vi "integrated_draft_1.vi"() -> ()   [LabVIEW 2014]
doc: "This VI demonstrates the individual configuration of settings in I/W, W/I, and continuous operation modes.\n\nThis VI is not meant to be used with infusion-only models. \n\nNotes:\n(1) If continuous mode is selected, infuse volumes/rates will be used."
uses:
  <vilib>/Motion/FlexMotion/CustomControls/CustomControls.llb/AxisOrVectorSpace To Configure.flx
  <vilib>/Motion/FlexMotion/FunctionsVIs/StartStopMotion.llb/Start Motion (8 axes).flx
  <vilib>/Motion/FlexMotion/FunctionsVIs/Trajectory.llb/Check Move Complete Status (8 axes).flx
  <vilib>/Motion/FlexMotion/FunctionsVIs/StartStopMotion.llb/Stop Motion (8 axes).flx
  <instrlib>/KD Scientific 2XX Series/KD Scientific 2XX Series.lvlib
  <vilib>/vision/NI_Vision_Development_Module.lvlib
panel:
  in  "stop 2":bool
  out "Voltage (V)":dbl=0.3869919147841388
  out "Force (grams)":dbl=0.3869919147841388
  out "Force Graph (g)":dynamicdata(graph)
  in  "Zero":dbl=-99.6 format="%#_13g"
  out "Load Cell Output (mV)":dynamicdata(graph)
  in  "stop (F)":bool
  out "Darta from Pressure Transducer":dynamicdata(graph) caption="data"
  out "Pressure Transducer Array":dbl[](array[numeric])
  in  "Displacement in mm":dbl
  in  "Velocity in mm/s":dbl
  out "Image":T1(plugin-control)
  out "Particle Measurements (Pixels) (Particle Analysis 1)":dbl[][](array[numeric]) format="%.2f"
  out "subarray":dbl[](array[numeric])
  out "The diameter":dbl[](array[numeric])
  out "Image from  Vision Acquisition 1":T1(plugin-control)
  out "Units":string
  out "Delivered Volume":dbl
  in  "stop":bool
  out "Status":T2
  in  "Baud Rate (9600)":u32(ring)=9600 items=["300"=300, "1200"=1200, "2400"=2400, "4800"=4800, "9600"=9600]
  in  "Withdrawal Settings":T3={"Flow Rate (5)"=5.0, "Volume (10)"=10.0, "Volume Units (ml)"=enum."milliliters (ml)", "Rate Units (ml/min.)"=enum."milliliters per minute (ml/min.)"} {"Volume (10)" format="%#.3g"}
  in  "Diameter (8.75 mm)":dbl=8.75
  in  "Infusion Settings":T3={"Flow Rate (5)"=5.0, "Volume (10)"=10.0, "Volume Units (ml)"=enum."milliliters (ml)", "Rate Units (ml/min.)"=enum."milliliters per minute (ml/min.)"}
  in  "Operation Mode (Infuse)":u16(ring) items=["Infuse", "Withdraw", "Infuse-Withdraw", "Withdraw-Infuse", "Continuous"]
  in  "Address (0)":i32 format="%0.0f"
  in  "error in (no error)":errorcluster
  in  "VISA resource name":refnum<visa-resource-name>="COM1"
  # "CCD Camera Input"
  # "Load Cell Input"
  # "Syringe Pump Control"
  # "RS-232 Settings"
  # "General Settings"
  # "Pump Status"
  # "Pressure Transducer"
  # "Displacement Motor Control"
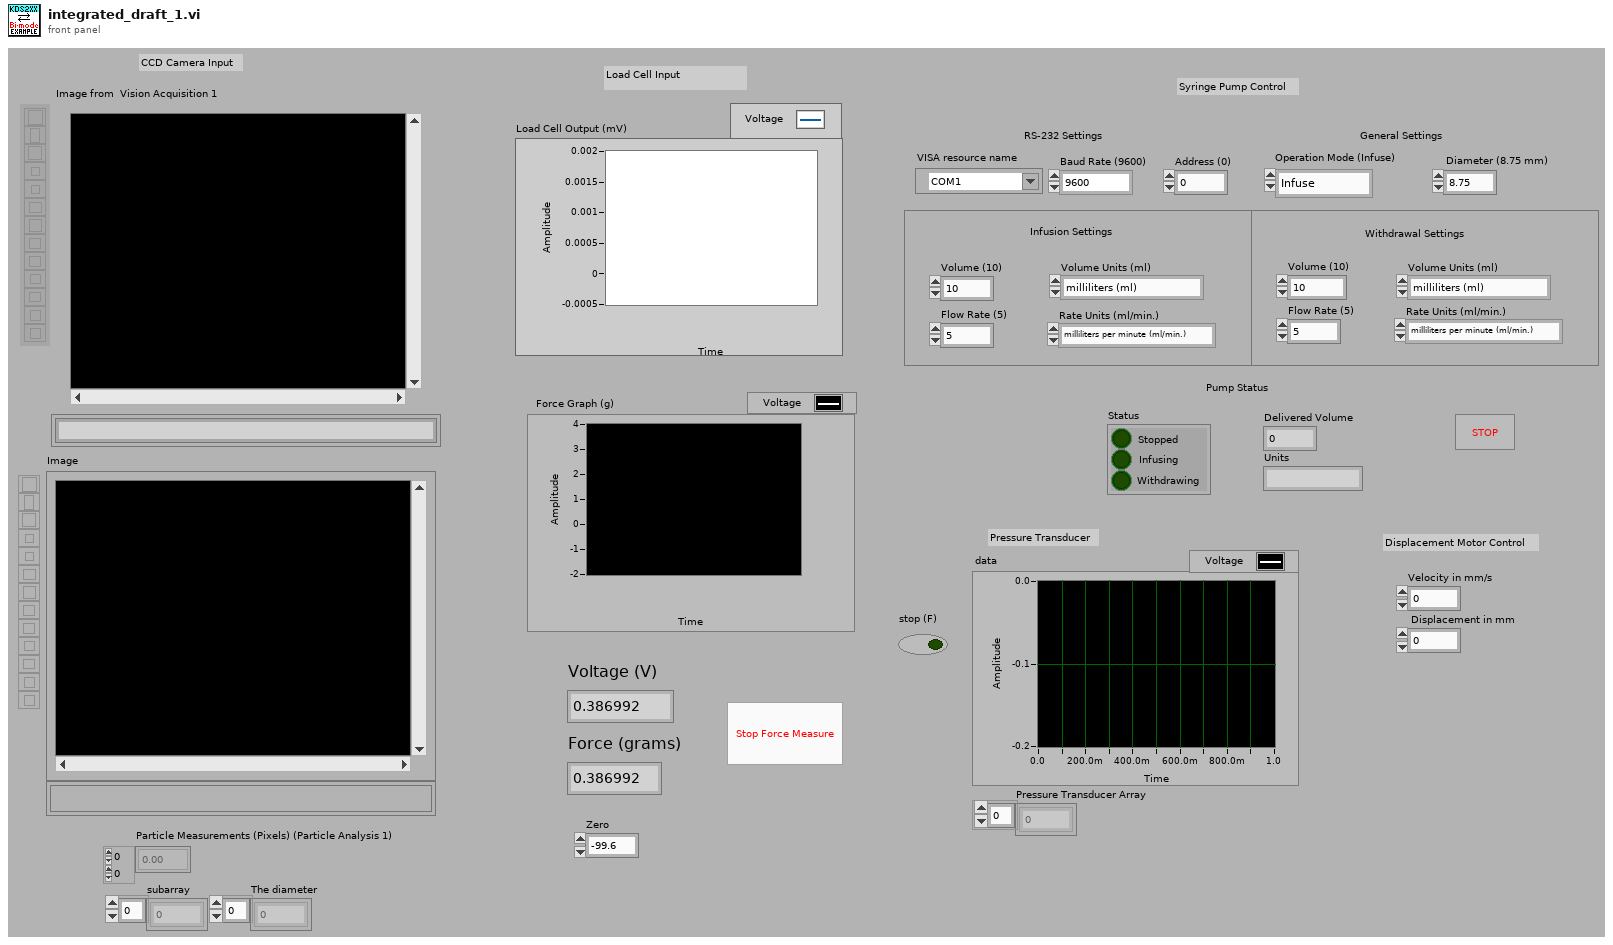
[diagram p1: front panel]
types:
  T1 = typedef "IMAQ Image.ctl" = refnum<image>
  T2 = cluster{"Stopped":bool, "Infusing":bool, "Withdrawing":bool}
  T3 = cluster{"Flow Rate (5)":dbl, "Volume (10)":dbl, "Volume Units (ml)":enum16{"milliliters (ml)", "microliters (ul)"}, "Rate Units (ml/min.)":enum16{"milliliters per minute (ml/min.)", "milliliters per hour (ml/hr.)", "microliters per minute (ul/min.)", "microliters per hour (ul/hr.)"}}
  T4 = typedef "Board Id" = u8
  T5 = enum16{"Absolute Position", "Relative Position", "Velocity", "Relative to Cap Pos", "Modulus Position", "Absolute Contouring", "Relative Contouring"}
  T6 = typedef "ROI Descriptor" = cluster{"Global Rectangle":i32[], "Contours":cluster{"ID":enum32{"External", "Internal"}, "Type":u32, "Coordinates":i32[]}[]}
  T7 = typedef "AxisOrVectorSpace To Configure.flx" = u16
  T8 = typedef "Resource Out (Enum).flx" = u16
  T9 = typedef "Bd Id Out" = u8
  T10 = enum16{"milliliters per minute (ml/min.)", "milliliters per hour (ml/hr.)", "microliters per minute (ul/min.)", "microliters per hour (ul/hr.)"}
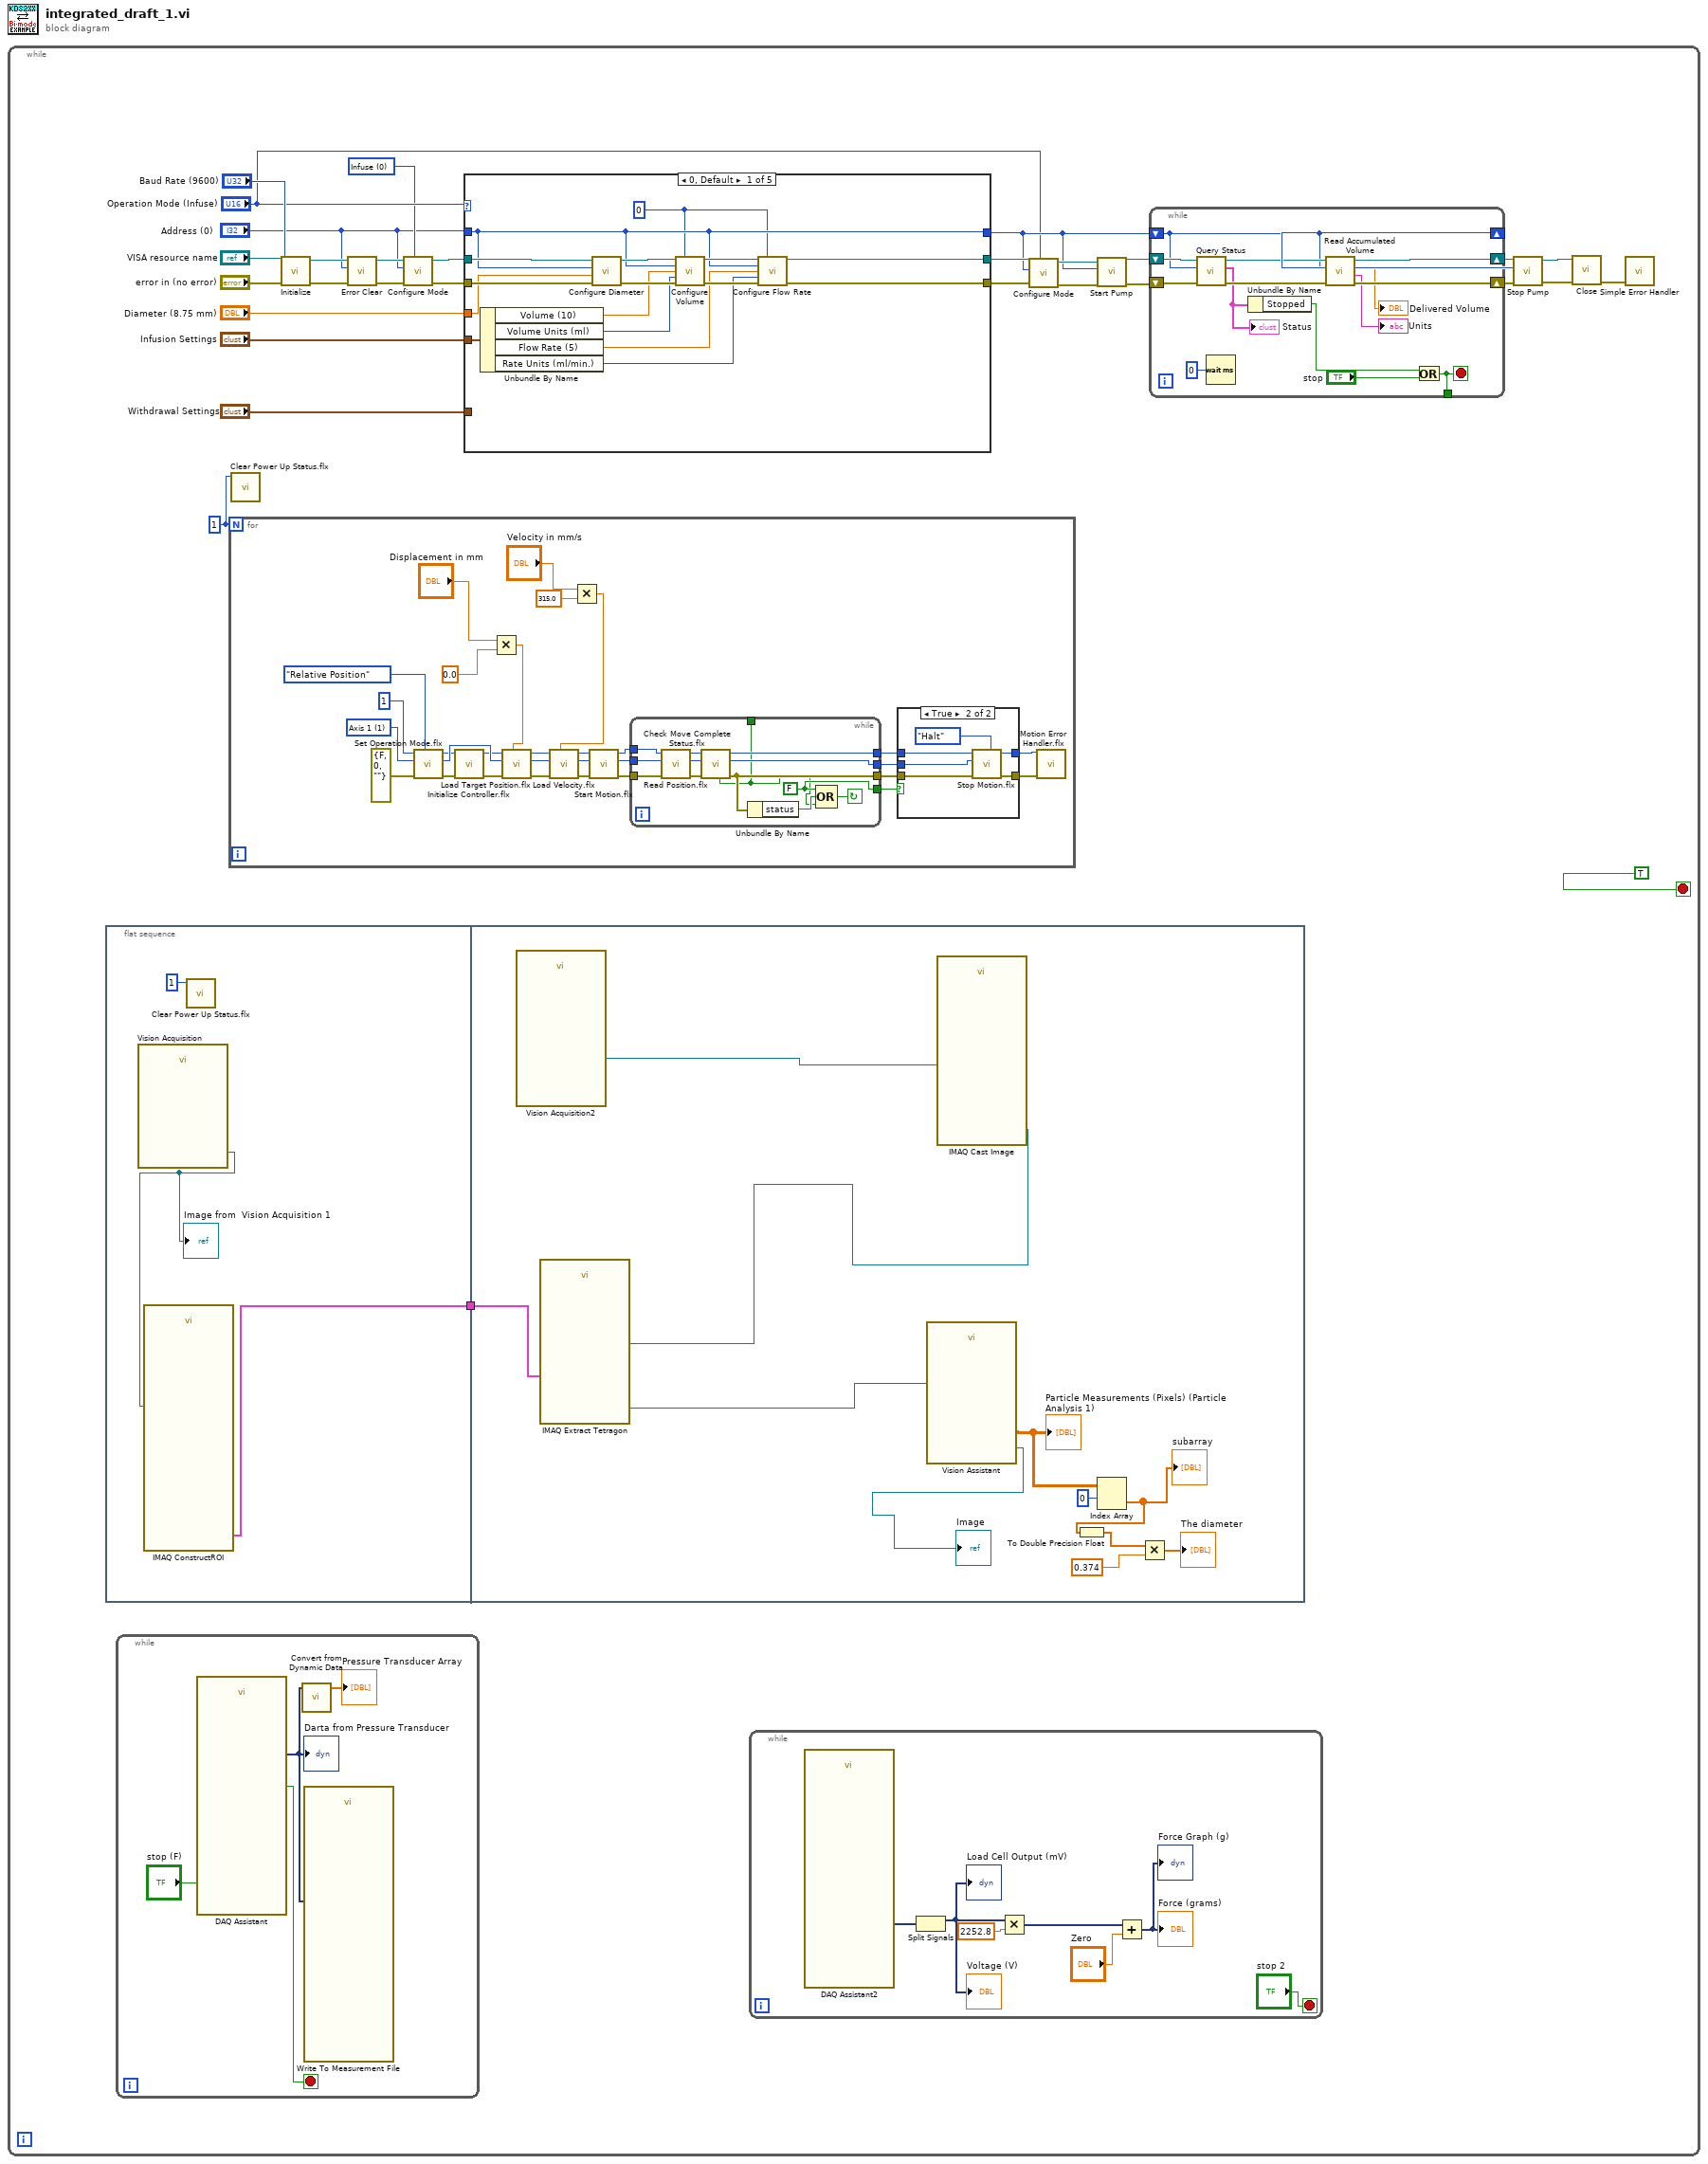
[diagram p0: block diagram]
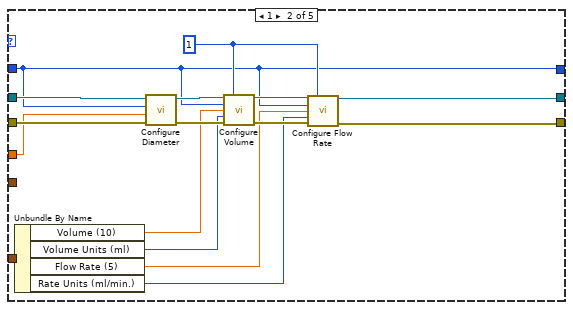
[diagram p3: hidden frame]
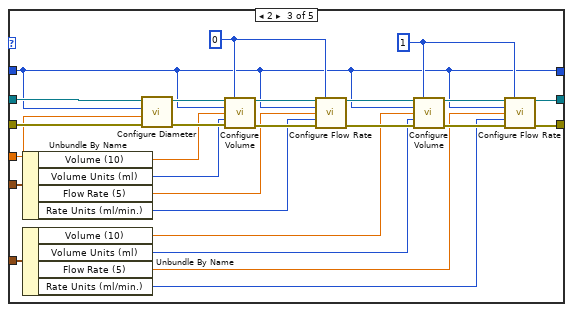
[diagram p4: hidden frame]
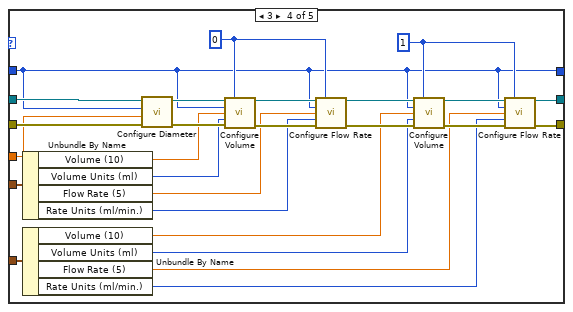
[diagram p5: hidden frame]
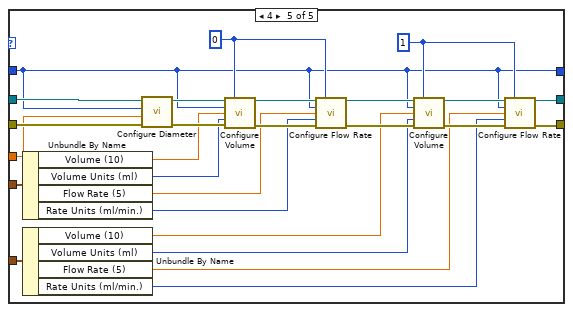
[diagram p6: hidden frame]
diagram:
  n1 = while {
    stop <- TRUE stop-if-true
    w3 = T4 1 ("Board ID")
    w9 = u16 0 items=["Infuse", "Withdraw", "Infuse-Withdraw", "Withdraw-Infuse", "Continuous"] ("Mode (infuse)")
    n2 = flat-sequence {
      tunnel: [w45] -> w1
      tunnel: w1 -> [w56]
      frame #0 {
        n3 = call "Vision Acquisition"() -> ("Image Out"=w43:T1)  [unwired: 26 in, 1 out]
        "Image from  Vision Acquisition 1" <- w43
        n4 = call "IMAQ ConstructROI"("Image"=w43) -> ("ROI Descriptor Out"=w45:T6)  [unwired: 7 in, 3 out]
        n5 = call <vilib>:"Clear Power Up Status.flx"("Board ID"=T4 1) -> ()  [unwired: 6 in, 2 out]
      }
      frame #1 {
        n6 = call "Vision Acquisition2"() -> ("Image Out"=w54:T1)  [unwired: 25 in, 2 out]
        n7 = call "IMAQ Cast Image"("Image Src"=w54) -> ("Image Dst Out"=w52:T1)  [unwired: 9 in, 1 out]
        n8 = call-poly "IMAQ Extract Tetragon"("ROI Descriptor"=w56, "Image Src"=w52) -> ("Image Dst Out"=w53:T1)  [unwired: 8 in, 1 out]
        n9 = call "Vision Assistant"("Image In"=w53) -> ("Image Out"=→"Image":T1, "Particle Measurements (Pixels) (Particle Analysis 1)"=w51:dbl[][])  [unwired: 23 in, 2 out]
        "Particle Measurements (Pixels) (Particle Analysis 1)" <- w51
        n10 = Index Array(array=w51, index (row)=0) -> (element=w49:dbl[])  [unwired: 1 in]
        "subarray" <- w49
        n11 = To Double Precision Float(number=w49) -> (double precision float=w48:dbl[])
        n12 = Multiply(x=w48, y=0.374) -> (x*y=→"The diameter":dbl[])
      }
    }
    n13 = while {
      stop <- w41 stop-if-true
      n14 = call "DAQ Assistant"("stop (F)"="stop (F)") -> ("data"=w39:dynamicdata, "stopped"=w41:bool)  [unwired: 15 in, 2 out]
      "Darta from Pressure Transducer" <- w39
      n15 = call "Convert from Dynamic Data"("Dynamic Data Type"=w39) -> ("Array"=→"Pressure Transducer Array":dbl[])  [unwired: 3 in]
      n16 = call "Write To Measurement File"("Signals"=w39) -> ()  [unwired: 16 in, 3 out]
    }
    n17 = for {
      N: w3 -> [_]
      w84 = T7 1 items=["Axis 1"=1, "Axis 2"=2, "Axis 3"=3, "Axis 4"=4, "Axis 5"=5, "Axis 6"=6, "Axis 7"=7, "Axis 8"=8, "Vector Space 1"=17, "Vector Space 2"=18, "Vector Space 3"=19, "Vector Space 4"=20] ("Axis or Vector Space")
      n18 = call <vilib>:"Set Operation Mode.flx"("Position Mode (Absolute)"=T5."Relative Position", "error in (no error)"=errorcluster {"status"=FALSE, "code"=0, "source"=""} ("error constant"), "Axis or Vector Space"=w84, "Board ID"=T4 1) -> ("error out"=w82:errorcluster, "Resource Output"=w81:T8, "Bd ID Out"=w80:T9)  [unwired: 2 in]
      n19 = call <vilib>:"Initialize Controller.flx"("error in (no error)"=w82, "Board ID"=w80) -> ("error out"=w75:errorcluster, "Bd ID Out"=w79:T9)  [unwired: 6 in]
      n20 = Multiply(x="Displacement in mm", y=0.0) -> (x*y=w59:dbl)
      n21 = call <vilib>:"Load Target Position.flx"("Target Position (0)"=w59, "error in (no error)"=w75, "Axis"=w81, "Board ID"=w79) -> ("error out"=w76:errorcluster, "Resource Output"=w77:T8, "Bd ID Out"=w78:T9)  [unwired: 3 in]
      n22 = Multiply(x="Velocity in mm/s", y=315.0) -> (x*y=w60:dbl)
      n23 = call <vilib>:"Load Velocity.flx"("Velocity (10000)"=w60, "error in (no error)"=w76, "Axis or Vector Space"=w77, "Board ID"=w78) -> ("error out"=w72:errorcluster, "Resource Output"=w73:T8, "Bd ID Out"=w74:T9)  [unwired: 3 in]
      n24 = call-poly <vilib>:"Start Motion.flx"("error in (no error)"=w72, "Axis or Vector Space"=w73, "Board ID"=w74) -> ("error out"=w69:errorcluster, "Resource Output"=w70:T8, "Bd ID Out"=w71:T9)  [unwired: 3 in]
      n25 = while {
        tunnel: w71 -> [w107]
        tunnel: w70 -> [w106]
        tunnel: w69 -> [w105]
        tunnel: [w100] -> w68
        tunnel: [w99] -> w67
        tunnel: [w97] -> w66
        tunnel: [w96] -> w65
        tunnel: [w95] -> _
        stop <- w101 continue-if-true
        w100 = FALSE
        n26 = call <vilib>:"Read Position.flx"("error in (no error)"=w105, "Axis"=w106, "Board ID"=w107) -> ("error out"=w102:errorcluster, "Resource Output"=w103:T8, "Bd ID Out"=w104:T9)  [unwired: 3 in, 1 out]
        n27 = call-poly <vilib>:"Check Move Complete Status.flx"("error in (no error)"=w102, "Axis or Vector Space"=w103, "Board ID"=w104) -> ("error out"=w99:errorcluster, "Resource Output"=w96:T8, "Bd ID Out"=w97:T9, "Move Complete"=w95:bool)  [unwired: 3 in]
        n28 = Unbundle By Name(w99) -> ("status"=w98:bool)
        n29 = Compound Arithmetic op=OR(w100, w98, w95) -> (w101:bool)
      }
      n30 = case shown="True" w68 {
        tunnel: w67 -> [w87 w93]
        tunnel: w66 -> [w88 w92]
        tunnel: w65 -> [_ w91]
        tunnel: [w87 w90] -> w64
        tunnel: [w88 w89] -> w63
        frame False {
        }
        frame True {
          n31 = call-poly <vilib>:"Stop Motion.flx"("Stop Type (Decel)"=enum16{"Decelerate", "Halt", "Kill"}."Halt", "error in (no error)"=w93, "Axis or Vector Space"=w91, "Board ID"=w92) -> ("error out"=w90:errorcluster, "Bd ID Out"=w89:T9)  [unwired: 3 in, 1 out]
        }
      }
      n32 = call <vilib>:"Motion Error Handler.flx"("Board ID"=w63, "error in (no error)"=w64) -> ()  [unwired: 9 in, 5 out]
    }
    n33 = call <vilib>:"Clear Power Up Status.flx"("Board ID"=w3) -> ()  [unwired: 6 in, 2 out]
    n34 = call <instrlib>:"Initialize.vi"("error in (no error)"="error in (no error)", "Baud Rate (9600)"="Baud Rate (9600)", "VISA resource name"="VISA resource name") -> ("error out"=w6:errorcluster, "VISA resource name out"=w5:refnum<visa-resource-name>)  [unwired: 7 in]
    n35 = call <instrlib>:"Error Clear.vi"("error in (no error)"=w6, "Address (0)"="Address (0)", "VISA resource name"=w5) -> ("error out"=w7:errorcluster, "VISA resource name out"=w8:refnum<visa-resource-name>)  [unwired: 6 in, 1 out]
    n36 = call <instrlib>:"Configure Mode.vi"("Mode (infuse)"=w9, "error in (no error)"=w7, "Address (0)"="Address (0)", "VISA resource name"=w8) -> ("error out"=w11:errorcluster, "VISA resource name out"=w10:refnum<visa-resource-name>)  [unwired: 6 in]
    n37 = case shown="0, Default" "Operation Mode (Infuse)" {
      tunnel: "Infusion Settings" -> [w117 _ w165 w191 w217]
      tunnel: "Withdrawal Settings" -> [_ w139 w164 w190 w216]
      tunnel: w10 -> [w123 w138 w163 w189 w215]
      tunnel: w11 -> [w122 w134 w162 w188 w214]
      tunnel: "Diameter (8.75 mm)" -> [w116 w130 w145 w171 w197]
      tunnel: [w115 w124 w140 w166 w192] -> w13
      tunnel: "Address (0)" -> [w115 w124 w140 w166 w192]
      tunnel: [w110 w135 w142 w168 w194] -> w17
      tunnel: [w109 w131 w141 w167 w193] -> w16
      frame 0, Default {
        w108 = 0
        n38 = Unbundle By Name(w117) -> ("Volume (10)"=w114:dbl, "Volume Units (ml)"=w113:enum16{"milliliters (ml)", "microliters (ul)"}, "Flow Rate (5)"=w112:dbl, "Rate Units (ml/min.)"=w111:T10)
        n39 = call <instrlib>:"Configure Diameter.vi"("error in (no error)"=w122, "Diameter (8.75 mm)"=w116, "Address (0)"=w115, "VISA resource name"=w123) -> ("error out"=w120:errorcluster, "VISA resource name out"=w121:refnum<visa-resource-name>)  [unwired: 6 in]
        n40 = call <instrlib>:"Configure Volume.vi"("VISA resource name"=w121, "Mode (infuse)"=w108, "Address (0)"=w115, "Volume (100)"=w114, "Units (0: milliliters)"=w113, "error in (no error)"=w120) -> ("VISA resource name out"=w119:refnum<visa-resource-name>, "error out"=w118:errorcluster)  [unwired: 8 in]
        n41 = call <instrlib>:"Configure Flow Rate.vi"("VISA resource name"=w119, "Mode (infuse)"=w108, "Address (0)"=w115, "Flow Rate (5)"=w112, "Units (0: milliliters per minute)"=w111, "error in (no error)"=w118) -> ("VISA resource name out"=w110:refnum<visa-resource-name>, "error out"=w109:errorcluster)  [unwired: 8 in]
      }
      frame 1 {
        w125 = 1
        n42 = Unbundle By Name(w139) -> ("Volume (10)"=w129:dbl, "Volume Units (ml)"=w128:enum16{"milliliters (ml)", "microliters (ul)"}, "Flow Rate (5)"=w127:dbl, "Rate Units (ml/min.)"=w126:T10)
        n43 = call <instrlib>:"Configure Diameter.vi"("error in (no error)"=w134, "Diameter (8.75 mm)"=w130, "Address (0)"=w124, "VISA resource name"=w138) -> ("error out"=w133:errorcluster, "VISA resource name out"=w137:refnum<visa-resource-name>)  [unwired: 6 in]
        n44 = call <instrlib>:"Configure Volume.vi"("VISA resource name"=w137, "Mode (infuse)"=w125, "Address (0)"=w124, "Volume (100)"=w129, "Units (0: milliliters)"=w128, "error in (no error)"=w133) -> ("VISA resource name out"=w136:refnum<visa-resource-name>, "error out"=w132:errorcluster)  [unwired: 8 in]
        n45 = call <instrlib>:"Configure Flow Rate.vi"("VISA resource name"=w136, "Mode (infuse)"=w125, "Address (0)"=w124, "Flow Rate (5)"=w127, "Units (0: milliliters per minute)"=w126, "error in (no error)"=w132) -> ("VISA resource name out"=w135:refnum<visa-resource-name>, "error out"=w131:errorcluster)  [unwired: 8 in]
      }
      frame 2 {
        w143 = 1
        w144 = 0
        n46 = Unbundle By Name(w165) -> ("Volume (10)"=w153:dbl, "Volume Units (ml)"=w152:enum16{"milliliters (ml)", "microliters (ul)"}, "Flow Rate (5)"=w151:dbl, "Rate Units (ml/min.)"=w150:T10)
        n47 = Unbundle By Name(w164) -> ("Volume (10)"=w149:dbl, "Volume Units (ml)"=w148:enum16{"milliliters (ml)", "microliters (ul)"}, "Flow Rate (5)"=w147:dbl, "Rate Units (ml/min.)"=w146:T10)
        n48 = call <instrlib>:"Configure Diameter.vi"("error in (no error)"=w162, "Diameter (8.75 mm)"=w145, "Address (0)"=w140, "VISA resource name"=w163) -> ("error out"=w157:errorcluster, "VISA resource name out"=w161:refnum<visa-resource-name>)  [unwired: 6 in]
        n49 = call <instrlib>:"Configure Volume.vi"("VISA resource name"=w161, "Mode (infuse)"=w144, "Address (0)"=w140, "Volume (100)"=w153, "Units (0: milliliters)"=w152, "error in (no error)"=w157) -> ("VISA resource name out"=w160:refnum<visa-resource-name>, "error out"=w156:errorcluster)  [unwired: 8 in]
        n50 = call <instrlib>:"Configure Flow Rate.vi"("VISA resource name"=w160, "Mode (infuse)"=w144, "Address (0)"=w140, "Flow Rate (5)"=w151, "Units (0: milliliters per minute)"=w150, "error in (no error)"=w156) -> ("VISA resource name out"=w159:refnum<visa-resource-name>, "error out"=w155:errorcluster)  [unwired: 8 in]
        n51 = call <instrlib>:"Configure Volume.vi"("VISA resource name"=w159, "Mode (infuse)"=w143, "Address (0)"=w140, "Volume (100)"=w149, "Units (0: milliliters)"=w148, "error in (no error)"=w155) -> ("VISA resource name out"=w158:refnum<visa-resource-name>, "error out"=w154:errorcluster)  [unwired: 8 in]
        n52 = call <instrlib>:"Configure Flow Rate.vi"("VISA resource name"=w158, "Mode (infuse)"=w143, "Address (0)"=w140, "Flow Rate (5)"=w147, "Units (0: milliliters per minute)"=w146, "error in (no error)"=w154) -> ("VISA resource name out"=w142:refnum<visa-resource-name>, "error out"=w141:errorcluster)  [unwired: 8 in]
      }
      frame 3 {
        w169 = 1
        w170 = 0
        n53 = Unbundle By Name(w191) -> ("Volume (10)"=w179:dbl, "Volume Units (ml)"=w178:enum16{"milliliters (ml)", "microliters (ul)"}, "Flow Rate (5)"=w177:dbl, "Rate Units (ml/min.)"=w176:T10)
        n54 = Unbundle By Name(w190) -> ("Volume (10)"=w175:dbl, "Volume Units (ml)"=w174:enum16{"milliliters (ml)", "microliters (ul)"}, "Flow Rate (5)"=w173:dbl, "Rate Units (ml/min.)"=w172:T10)
        n55 = call <instrlib>:"Configure Diameter.vi"("error in (no error)"=w188, "Diameter (8.75 mm)"=w171, "Address (0)"=w166, "VISA resource name"=w189) -> ("error out"=w183:errorcluster, "VISA resource name out"=w187:refnum<visa-resource-name>)  [unwired: 6 in]
        n56 = call <instrlib>:"Configure Volume.vi"("VISA resource name"=w187, "Mode (infuse)"=w170, "Address (0)"=w166, "Volume (100)"=w179, "Units (0: milliliters)"=w178, "error in (no error)"=w183) -> ("VISA resource name out"=w186:refnum<visa-resource-name>, "error out"=w182:errorcluster)  [unwired: 8 in]
        n57 = call <instrlib>:"Configure Flow Rate.vi"("VISA resource name"=w186, "Mode (infuse)"=w170, "Address (0)"=w166, "Flow Rate (5)"=w177, "Units (0: milliliters per minute)"=w176, "error in (no error)"=w182) -> ("VISA resource name out"=w185:refnum<visa-resource-name>, "error out"=w181:errorcluster)  [unwired: 8 in]
        n58 = call <instrlib>:"Configure Volume.vi"("VISA resource name"=w185, "Mode (infuse)"=w169, "Address (0)"=w166, "Volume (100)"=w175, "Units (0: milliliters)"=w174, "error in (no error)"=w181) -> ("VISA resource name out"=w184:refnum<visa-resource-name>, "error out"=w180:errorcluster)  [unwired: 8 in]
        n59 = call <instrlib>:"Configure Flow Rate.vi"("VISA resource name"=w184, "Mode (infuse)"=w169, "Address (0)"=w166, "Flow Rate (5)"=w173, "Units (0: milliliters per minute)"=w172, "error in (no error)"=w180) -> ("VISA resource name out"=w168:refnum<visa-resource-name>, "error out"=w167:errorcluster)  [unwired: 8 in]
      }
      frame 4 {
        w195 = 1
        w196 = 0
        n60 = Unbundle By Name(w217) -> ("Volume (10)"=w205:dbl, "Volume Units (ml)"=w204:enum16{"milliliters (ml)", "microliters (ul)"}, "Flow Rate (5)"=w203:dbl, "Rate Units (ml/min.)"=w202:T10)
        n61 = Unbundle By Name(w216) -> ("Volume (10)"=w201:dbl, "Volume Units (ml)"=w200:enum16{"milliliters (ml)", "microliters (ul)"}, "Flow Rate (5)"=w199:dbl, "Rate Units (ml/min.)"=w198:T10)
        n62 = call <instrlib>:"Configure Diameter.vi"("error in (no error)"=w214, "Diameter (8.75 mm)"=w197, "Address (0)"=w192, "VISA resource name"=w215) -> ("error out"=w209:errorcluster, "VISA resource name out"=w213:refnum<visa-resource-name>)  [unwired: 6 in]
        n63 = call <instrlib>:"Configure Volume.vi"("VISA resource name"=w213, "Mode (infuse)"=w196, "Address (0)"=w192, "Volume (100)"=w205, "Units (0: milliliters)"=w204, "error in (no error)"=w209) -> ("VISA resource name out"=w212:refnum<visa-resource-name>, "error out"=w208:errorcluster)  [unwired: 8 in]
        n64 = call <instrlib>:"Configure Flow Rate.vi"("VISA resource name"=w212, "Mode (infuse)"=w196, "Address (0)"=w192, "Flow Rate (5)"=w203, "Units (0: milliliters per minute)"=w202, "error in (no error)"=w208) -> ("VISA resource name out"=w211:refnum<visa-resource-name>, "error out"=w207:errorcluster)  [unwired: 8 in]
        n65 = call <instrlib>:"Configure Volume.vi"("VISA resource name"=w211, "Mode (infuse)"=w195, "Address (0)"=w192, "Volume (100)"=w201, "Units (0: milliliters)"=w200, "error in (no error)"=w207) -> ("VISA resource name out"=w210:refnum<visa-resource-name>, "error out"=w206:errorcluster)  [unwired: 8 in]
        n66 = call <instrlib>:"Configure Flow Rate.vi"("VISA resource name"=w210, "Mode (infuse)"=w195, "Address (0)"=w192, "Flow Rate (5)"=w199, "Units (0: milliliters per minute)"=w198, "error in (no error)"=w206) -> ("VISA resource name out"=w194:refnum<visa-resource-name>, "error out"=w193:errorcluster)  [unwired: 8 in]
      }
    }
    n67 = while {
      stop <- "stop 2" stop-if-true
      n68 = call "DAQ Assistant2"() -> ("data"=w37:dynamicdata)  [unwired: 16 in, 3 out]
      n69 = Split Signals(w37) -> (w32:dynamicdata)  [unwired: 2 in, 1 out]
      "Voltage (V)" <- w32
      "Load Cell Output (mV)" <- w32
      n70 = Multiply(x=w32, y=2252.8) -> (x*y=w36:dynamicdata)
      n71 = Add(x=w36, y="Zero") -> (x+y=→"Force (grams)" →"Force Graph (g)":dynamicdata)
    }
    n72 = call <instrlib>:"Configure Mode.vi"("Mode (infuse)"="Operation Mode (Infuse)", "error in (no error)"=w16, "Address (0)"=w13, "VISA resource name"=w17) -> ("error out"=w14:errorcluster, "VISA resource name out"=w15:refnum<visa-resource-name>)  [unwired: 6 in]
    n73 = call <instrlib>:"Start Pump.vi"("error in (no error)"=w14, "Address (0)"=w13, "VISA resource name"=w15) -> ("error out"=w28:errorcluster, "VISA resource name out"=w29:refnum<visa-resource-name>)  [unwired: 7 in]
    n74 = while {
      shift-right: [w221] -> w22
      shift-left: w13 -> [w221]
      shift-right: [w223] -> w27
      shift-left: w29 -> [w228]
      shift-right: [w222] -> w26
      shift-left: w28 -> [w229]
      tunnel: [w218] -> _
      stop <- w218 stop-if-true
      n75 = call <instrlib>:"Query Status.vi"("error in (no error)"=w229, "Address (0)"=w221, "VISA resource name"=w228) -> ("error out"=w231:errorcluster, "Status"=w227:T2, "VISA resource name out"=w224:refnum<visa-resource-name>)  [unwired: 6 in]
      "Status" <- w227
      n76 = Wait (ms)(milliseconds to wait=u32 0) -> ()  [unwired: 1 out]
      n77 = Unbundle By Name(w227) -> ("Stopped"=w226:bool)
      n78 = call <instrlib>:"Read Accumulated Volume.vi"("error in (no error)"=w231, "Address (0)"=w221, "VISA resource name"=w224) -> ("error out"=w222:errorcluster, "Units"=→"Units":string, "Delivered Volume"=→"Delivered Volume":dbl, "VISA resource name out"=w223:refnum<visa-resource-name>)  [unwired: 5 in]
      n79 = Or(x=w226, y="stop") -> (x .or. y?=w218:bool)
    }
    n80 = call <instrlib>:"Stop Pump.vi"("error in (no error)"=w26, "Address (0)"=w22, "VISA resource name"=w27) -> ("error out"=w20:errorcluster, "VISA resource name out"=w19:refnum<visa-resource-name>)  [unwired: 7 in]
    n81 = call <instrlib>:"Close.vi"("error in (no error)"=w20, "VISA resource name"=w19) -> ("error out"=w21:errorcluster)  [unwired: 9 in]
    n82 = call <vilib>:"Simple Error Handler.vi"("error in (no error)"=w21) -> ()  [unwired: 4 in, 5 out]
  }
